vi "Error Channels Write Single.vi"(8 "error in":errorcluster, 9 "Channel Index":i32, 10 "Error Channels STS":i32, 11 "Error Channels in":refnum<class "Error Channels.lvclass">) -> (0 "error out":errorcluster, 3 "Error Channels out":refnum<class "Error Channels.lvclass">)   [LabVIEW 2023, in "Error Channels.lvclass"]
uses:
  Error Channels.lvclass
  <vilib>/ADAS Replay HIL/Channels/Tag Wrapper/Tag Wrapper.lvlib
  <vilib>/ADAS Replay HIL/Channels/Tag Wrapper/Polymorphic/Write Channel (I32).vi
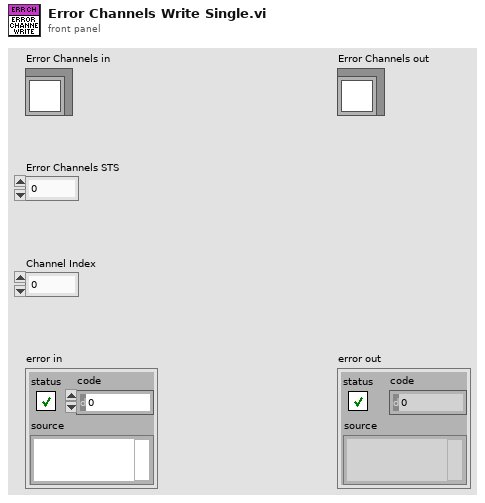
[diagram p1: front panel]
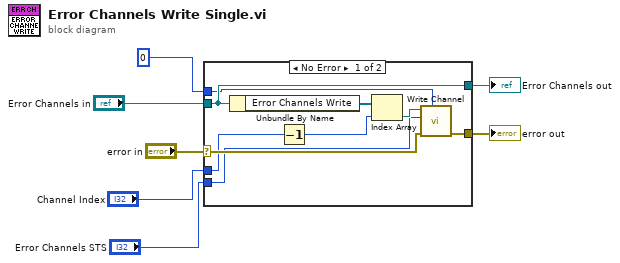
[diagram p0: block diagram]
diagram:
  n1 = case shown="No Error" "error in" {
    selector: "error in" -> [w16 w17]
    tunnel: [w15 w17] -> w4
    tunnel: [w10 w18] -> w6
    tunnel: "Error Channels in" -> [w10 w18]
    tunnel: "Channel Index" -> [w14 _]
    tunnel: "Error Channels STS" -> [w11 _]
    tunnel: 0 ("Timeout (ms)") -> [w8 _]
    frame No Error {
      n2 = Unbundle By Name(w10) -> ("Error Channels Write"=w9:refnum<k21>[])
      n3 = Decrement(x=w14) -> (x-1=w13:i32)
      n4 = Index Array(array=w9, index=w13) -> (element=w12:refnum<k21>)
      n5 = call-poly <vilib>:"Write Channel.vi"("Timeout (ms)"=w8, "error in"=w16, "Value to Write"=w11, "ADAS HIL Channel in"=w12) -> ("error out"=w15:errorcluster)  [unwired: 5 in, 2 out]
    }
    frame Error {
    }
  }
  "error out" <- w4
  "Error Channels out" <- w6
